vi "Change from Year to Version.vi"(11 "LabVIEW Year":dbl) -> (3 "LabVIEW Version Number":dbl)   [LabVIEW 2013]
doc: "Take the LabVIEW visible version and convert to internal version e.g. 8.6 is 8.6 or 2010 is 10.0"
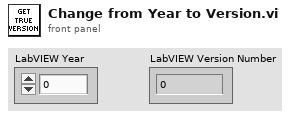
[diagram p1: front panel]
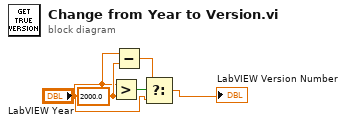
[diagram p0: block diagram]
diagram:
  w3 = 2000.0
  n1 = Greater?(x="LabVIEW Year", y=w3) -> (0:w1:bool)
  n2 = Subtract(x="LabVIEW Year", y=w3) -> (x-y=w4:dbl)
  n3 = Select(t=w4, s=w1, f="LabVIEW Year") -> (s? t:f=→"LabVIEW Version Number":dbl)
